vi "Squares.vi"() -> ()   [LabVIEW 2024]
panel:
  out "Numeric 2":dbl
  in  "Numeric":dbl
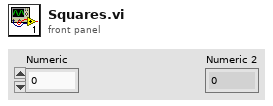
[diagram p1: front panel]
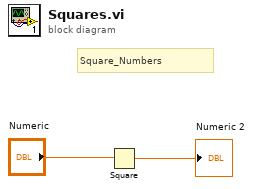
[diagram p0: block diagram]
diagram:
  # "Square_Numbers"
  n1 = Square(x="Numeric") -> (x^2=→"Numeric 2":dbl)
